vi "State_Machine.vi"(8 "error in (no error)":errorcluster caption="entrée d'erreur (pas d'erreur)", 11 "Nodon_ZCR_Delta_ON IN":refnum<class "Nodon_ZCR_Delta_ON.lvclass">) -> (0 "error out":errorcluster caption="sortie d'erreur", 2 "Json_String":string, 3 "Nodon_ZCR_Delta_ON Out":refnum<class "Nodon_ZCR_Delta_ON.lvclass">)   [LabVIEW 2020, in "Library Test.lvlib" / "Nodon_ZCR_Delta_ON.lvclass"]
uses:
  Nodon_ZCR_Delta_ON.lvclass
panel:
  out "String In progress":string
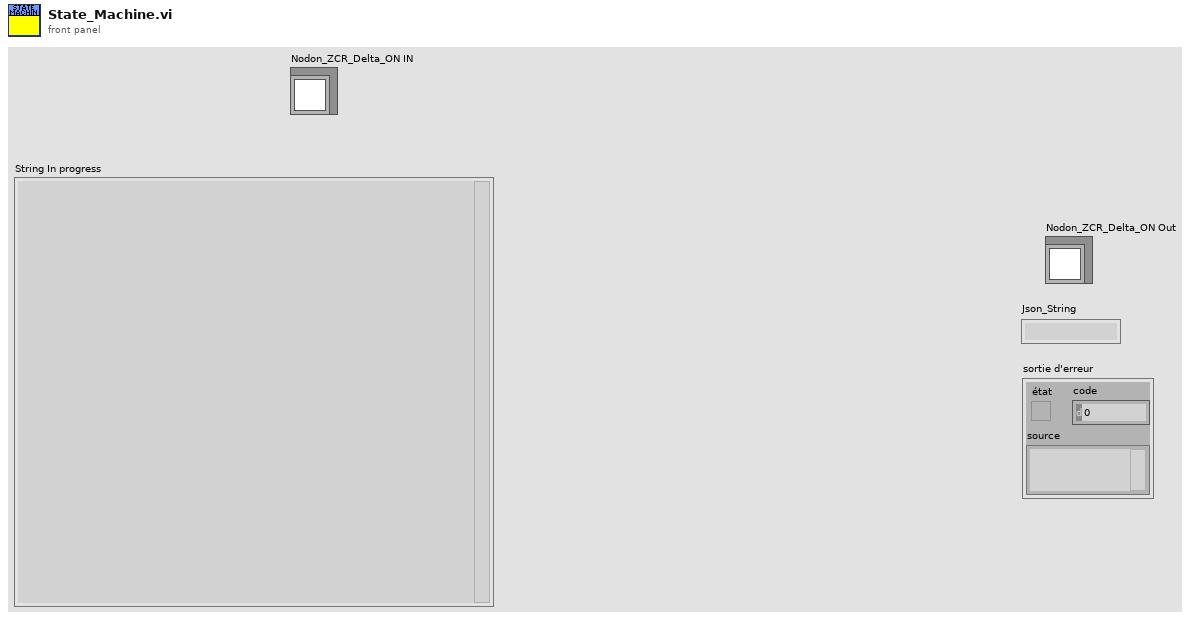
[diagram p1: front panel]
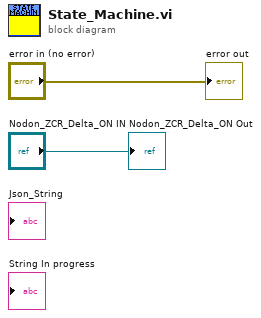
[diagram p0: block diagram]
diagram:
  "Nodon_ZCR_Delta_ON Out" <- "Nodon_ZCR_Delta_ON IN"
  "error out" <- "error in (no error)"
